vi "PreInit_must_call.vi"(6 "Open Actor Core front panel? (T)":bool=TRUE, 8 "error in (no error)":errorcluster, 11 "Mag Lab Measure Interface in":refnum<class "Mag Lab Measure UI.lvclass">) -> (0 "error out":errorcluster, 2 "stop event":refnum<user-event>, 3 "Mag Lab Measure Interface out":refnum<class "Mag Lab Measure UI.lvclass">)   [LabVIEW 2015, in "Mag Lab Measure UI.lvclass"]
uses:
  Mag Lab Measure UI.lvclass
  Mag Lab Root/Mag Lab Root.lvclass/Mag Lab Root.ctl
  Mag Lab Root/Write Front Panel ref.vi
  Mag Lab Root/Read Front Panel ref.vi
  Mag Lab Error Handler/Mag Lab Error Handler.lvclass
  Mag Lab Root/Mag Lab Root.lvclass
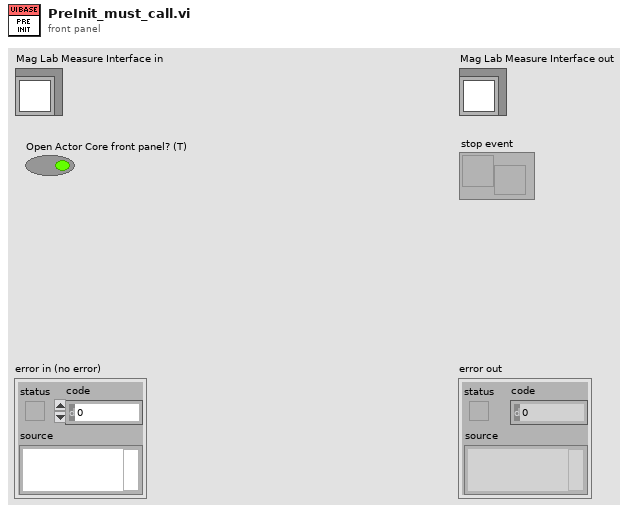
[diagram p1: front panel]
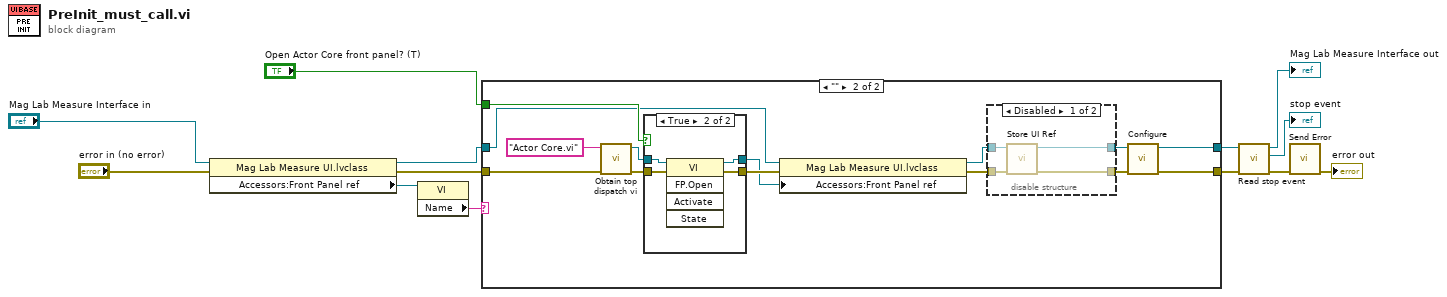
[diagram p0: block diagram]
diagram:
  n1 = property class="Mag Lab Measure UI.lvclass"(reference="Mag Lab Measure Interface in", error in="error in (no error)") -> (reference out=w1:refnum<class "Mag Lab Measure UI.lvclass">, error out=w2:errorcluster, "Accessors:Front Panel ref"=w4:refnum<vi>)
  n2 = property class="VI"(reference=w4) -> ("Name"=w13:string)  [unwired: 1 in, 2 out]
  n3 = case shown="\"\"" w13 {
    tunnel: [w15 w26] -> w9
    tunnel: w1 -> [w15 w17]
    tunnel: w2 -> [w14 w22]
    tunnel: [w14 w27] -> w10
    tunnel: "Open Actor Core front panel? (T)" -> [_ w28]
    frame Default {
    }
    frame "" {
      n4 = call "Obtain top dispatch vi.vi"("Error In"=w22, "VI name"="Actor Core.vi") -> ("Error Out"=w23:errorcluster, "vi reference"=w21:refnum<vi>)  [unwired: 7 in, 1 out]
      n5 = case shown="True" w28 {
        tunnel: w21 -> [w36 w41]
        tunnel: w23 -> [w37 w40]
        tunnel: [w37 w39] -> w29
        tunnel: [w36 w38] -> w16
        frame False {
        }
        frame True {
          n6 = invoke class="VI" method="FP.Open"(reference=w41, error in=w40) -> (reference out=w38:refnum<vi>, error out=w39:errorcluster)  [unwired: 3 in, 3 out]
        }
      }
      n7 = property class="Mag Lab Measure UI.lvclass"(reference=w17, error in=w29, "Accessors:Front Panel ref"=w16) -> (reference out=w25:refnum<class "Mag Lab Measure UI.lvclass">, error out=w24:errorcluster)
      n8 = disable-structure shown="Disabled" {
        disable-tunnel: w25 -> [w33 w35]
        disable-tunnel: [w32 w35] -> w18
        disable-tunnel: [w31 w34] -> w19
        disable-tunnel: w24 -> [w30 w34]
        frame Disabled {
          n9 = call "Store UI Ref.vi"("error in (no error)"=w30, "Mag Lab Measure Interface in"=w33) -> ("error out"=w31:errorcluster, "Mag Lab Measure Interface out"=w32:refnum<class "Mag Lab Measure UI.lvclass">)  [unwired: 8 in]
        }
        frame Enabled {
        }
      }
      n10 = call-dynamic "Configure.vi"("error in (no error)"=w19, "Mag Lab Measure Interface in"=w18) -> ("error out"=w27:errorcluster, "Mag Lab Measure Interface out"=w26:refnum<class "Mag Lab Measure UI.lvclass">)  [unwired: 8 in]
    }
  }
  n11 = call "Read stop event.vi"("error in (no error)"=w10, "Mag Lab Root in"=w9) -> ("error out"=w6:errorcluster, "stop event"=→"stop event":refnum<user-event>, "Mag Lab Root out"=→"Mag Lab Measure Interface out":refnum<class "Mag Lab Measure UI.lvclass">)  [unwired: 7 in]
  n12 = call "Send Error.vi"("error in (no error)"=w6) -> ("error out"=→"error out":errorcluster)  [unwired: 9 in, 1 out]
